vi "FVI_Trajectiore_Cercle.vi"(9 "Rayon y":dbl, 10 "Rayon x":dbl, 11 "dst":dbl) -> (0 "ARG":dbl(knob) scale=-180.0..180.0, 1 "ARD":dbl(knob) scale=-180.0..180.0, 2 "AVG":dbl(knob) scale=-180.0..180.0, 3 "AVD":dbl(knob) scale=-180.0..180.0)   [LabVIEW 2018]
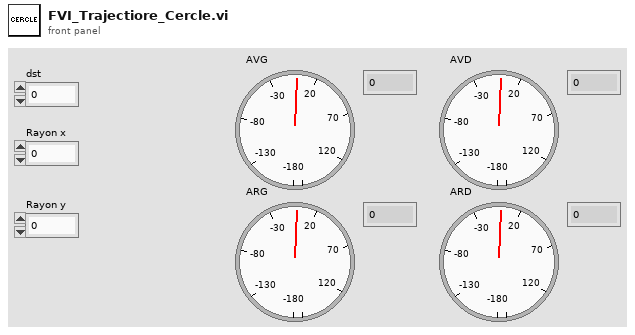
[diagram p1: front panel]
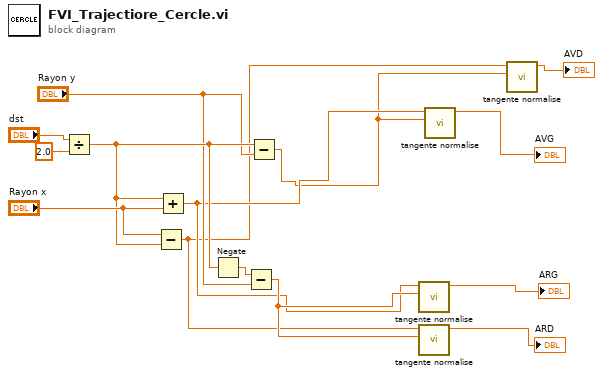
[diagram p0: block diagram]
diagram:
  n1 = Divide(x="dst", y=2.0) -> (x/y=w11:dbl)
  n2 = Subtract(x="Rayon x", y=w11) -> (x-y=w5:dbl)
  n3 = Add(x=w11, y="Rayon x") -> (x+y=w7:dbl)
  n4 = Negate(x=w11) -> (-x=w10:dbl)
  n5 = Subtract(x=w10, y="Rayon y") -> (x-y=w8:dbl)
  n6 = Subtract(x=w11, y="Rayon y") -> (x-y=w6:dbl)
  n7 = call "tangente normalise.vi"("a"=w8, "b"=w7) -> ("angle"=→"ARG":dbl)  [unwired: 9 in]
  n8 = call "tangente normalise.vi"("a"=w8, "b"=w5) -> ("angle"=→"ARD":dbl)  [unwired: 9 in]
  n9 = call "tangente normalise.vi"("a"=w6, "b"=w7) -> ("angle"=→"AVG":dbl)  [unwired: 9 in]
  n10 = call "tangente normalise.vi"("a"=w6, "b"=w5) -> ("angle"=→"AVD":dbl)  [unwired: 9 in]
